vi "Square Root.vi"() -> ()   [LabVIEW 2018]
panel:
  out "error out":errorcluster
  in  "error in (no error)":errorcluster
  out "Squre root":dbl
  in  "Squre root input":dbl
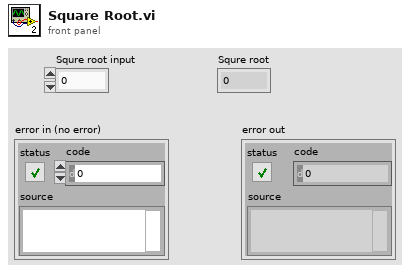
[diagram p1: front panel]
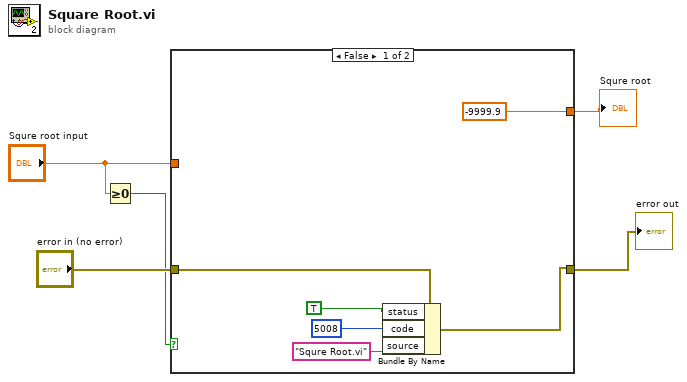
[diagram p0: block diagram]
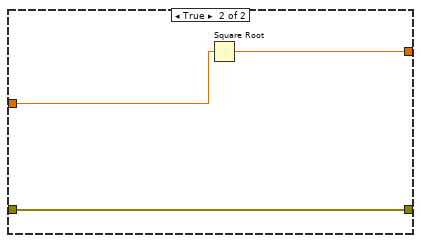
[diagram p2: hidden frame]
diagram:
  n1 = Greater Or Equal To 0?(x="Squre root input") -> (x >= 0?=w2:bool)
  n2 = case shown="False" w2 {
    tunnel: [-9999.9 w14] -> w5
    tunnel: "error in (no error)" -> [w10 w13]
    tunnel: [w9 w13] -> w3
    tunnel: "Squre root input" -> [_ w12]
    frame False {
      n3 = Bundle By Name(cluster=w10, "status"=TRUE, "code"=5008, "source"="Squre Root.vi") -> (w9:errorcluster)
    }
    frame True {
      n4 = Square Root(x=w12) -> (sqrt(x)=w14:dbl)
    }
  }
  "Squre root" <- w5
  "error out" <- w3
